vi "Set Parent Window(SubVI).vi"(8 "error in (no error)":errorcluster, 10 "Parent Name":string="TestSystem", 11 "Child Name":string="Numeric") -> (0 "error out":errorcluster, 3 "return type":i32)   [LabVIEW 2010]
uses:
  user32.dll
panel:
  out "return type 2":i32
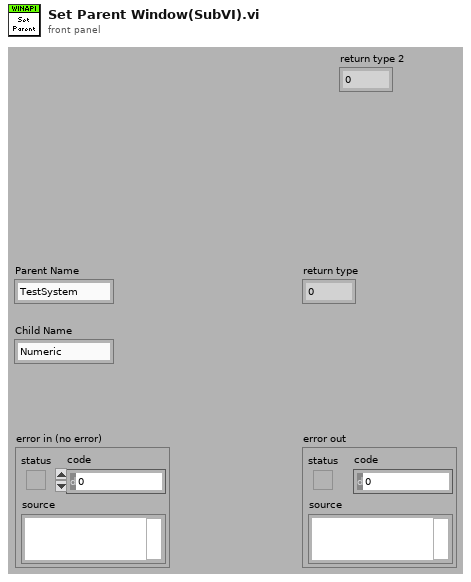
[diagram p1: front panel]
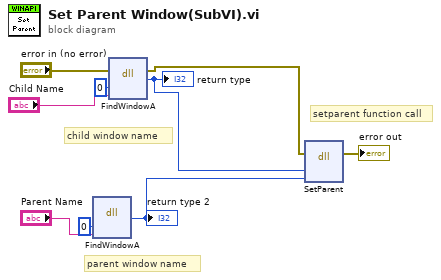
[diagram p0: block diagram]
diagram:
  # "setparent function call"
  # "child window name"
  # "parent window name"
  n1 = dll-call lib="user32.dll" fn="FindWindowA"("arg1"=0, "arg2"="Parent Name") -> ("return type"=w4:i32)  [unwired: 5 in, 2 out]
  "return type 2" <- w4
  n2 = dll-call lib="user32.dll" fn="FindWindowA"(error in="error in (no error)", "arg1"=0, "arg2"="Child Name") -> (error out=w1:errorcluster, "return type"=w5:i32)  [unwired: 4 in, 1 out]
  "return type" <- w5
  n3 = dll-call lib="user32.dll" fn="SetParent"(error in=w1, "arg1"=w5, "arg2"=w4) -> (error out=→"error out":errorcluster)  [unwired: 5 in, 1 out]
